vi "VRM Field Graphs.vi"(8 "error in (no error)":errorcluster, 10 "Target Field (T)":dbl[](array[numeric]), 11 "Field (T)":dbl[](array[numeric])) -> (0 "error out":errorcluster, 2 "XY Graph":cluster{dbl[], dbl[]}[](array[cluster]), 3 "XZ Graph":cluster{dbl[], dbl[]}[](array[cluster]))   [LabVIEW 2019, in "Instrument.OxfordVRM UI.lvclass"]
uses:
  Instrument.OxfordVRM UI.lvclass
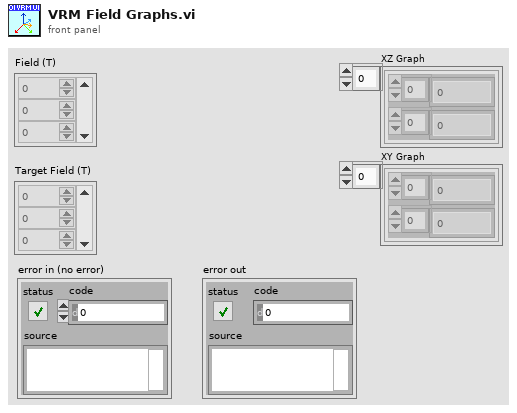
[diagram p1: front panel]
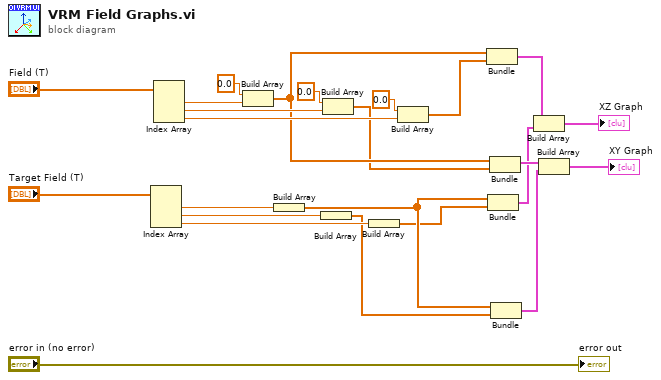
[diagram p0: block diagram]
diagram:
  n1 = Index Array(array="Target Field (T)") -> (element #1=w15:dbl, element #2=w14:dbl, element #3=w13:dbl)  [unwired: 3 in]
  n2 = Index Array(array="Field (T)") -> (element #1=w21:dbl, element #2=w16:dbl, element #3=w18:dbl)  [unwired: 3 in]
  n3 = Build Array(0.0 ("element"), w21) -> (w11:dbl[])
  n4 = Build Array(w15) -> (w5:dbl[])
  n5 = Build Array(w14) -> (w3:dbl[])
  n6 = Build Array(0.0 ("element"), w16) -> (w10:dbl[])
  n7 = Build Array(w13) -> (w4:dbl[])
  n8 = Build Array(0.0 ("element"), w18) -> (w12:dbl[])
  n9 = Bundle(w11, w12) -> (w9:cluster{dbl[], dbl[]})  [unwired: 1 in]
  n10 = Bundle(w5, w4) -> (w2:cluster{dbl[], dbl[]})  [unwired: 1 in]
  n11 = Bundle(w11, w10) -> (w8:cluster{dbl[], dbl[]})  [unwired: 1 in]
  n12 = Bundle(w5, w3) -> (w1:cluster{dbl[], dbl[]})  [unwired: 1 in]
  n13 = Build Array(w9, w2) -> (→"XZ Graph":cluster{dbl[], dbl[]}[])
  n14 = Build Array(w8, w1) -> (→"XY Graph":cluster{dbl[], dbl[]}[])
  "error out" <- "error in (no error)"
